vi "Read Region.vi"(8 "error in (no error)":errorcluster, 11 "AWS Core in":refnum<class "Bucket.lvclass">) -> (0 "error out":errorcluster, 2 "Region":T1, 3 "AWS Core out":refnum<class "Bucket.lvclass">)   [LabVIEW 2015, in "NI_AWS_S3.lvlib" / "Bucket.lvclass"]
uses:
  Bucket.lvclass
  Core/HTTP Request/Region.ctl
  Core/HTTP Request/HTTP Request.lvclass/HTTP Request.ctl
  Core/HTTP Request/Write Region.vi
  Core/HTTP Request/Read _regionSet.vi
  Core/HTTP Request/HTTP Request.lvclass
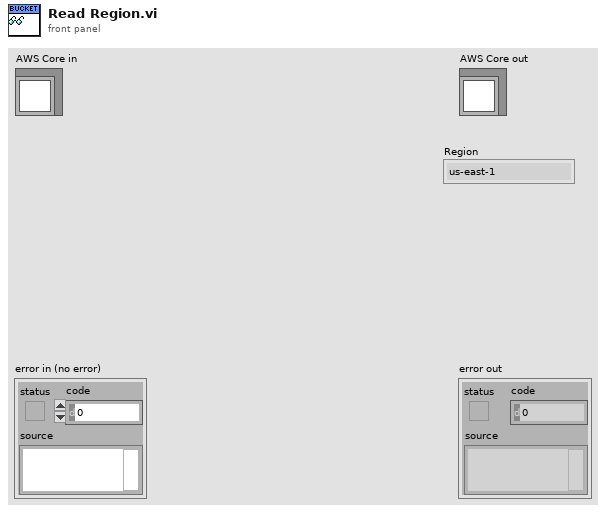
[diagram p1: front panel]
types:
  T1 = typedef "NI_AWS_Core.lvlib/HTTP Request.lvclass/Region.ctl" = enum16{"us-east-1", "us-east-2", "us-west-1", "us-west-2", "ap-northeast-1", "ap-northeast-2", "ap-southeast-1", "ap-southeast-2", "ca-central-1", "eu-central-1", "eu-west-1", "eu-west-2", "sa-east-1"}
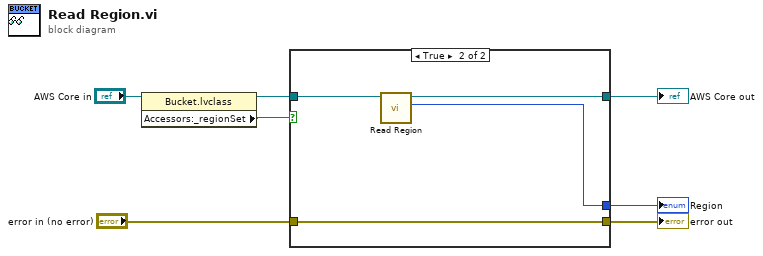
[diagram p0: block diagram]
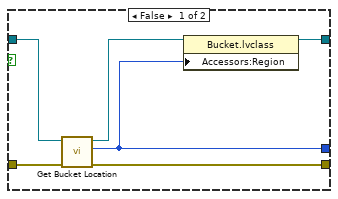
[diagram p2: hidden frame]
diagram:
  n1 = property class="Bucket.lvclass"(reference="AWS Core in") -> (reference out=w3:refnum<class "Bucket.lvclass">, "Accessors:_regionSet"=w4:bool)  [unwired: 1 in, 1 out]
  n2 = case shown="True" w4 {
    tunnel: "error in (no error)" -> [w13 w17]
    tunnel: [w12 w17] -> w5
    tunnel: [w11 w15] -> w2
    tunnel: w3 -> [w8 w16]
    tunnel: [w9 w14] -> w1
    frame False {
      n3 = call "Get Bucket Location.vi"("error in (no error)"=w13, "Bucket in"=w8) -> ("error out"=w12:errorcluster, "Location"=w9:T1, "Bucket out"=w10:refnum<class "Bucket.lvclass">)  [unwired: 7 in]
      n4 = property class="Bucket.lvclass"(reference=w10, "Accessors:Region"=w9) -> (reference out=w11:refnum<class "Bucket.lvclass">)  [unwired: 1 in, 1 out]
    }
    frame True {
      n5 = call-parent "Read Region.vi"("AWS Core in"=w16) -> ("Region"=w14:T1, "AWS Core out"=w15:refnum<class "Bucket.lvclass">)  [unwired: 8 in, 1 out]
    }
  }
  "error out" <- w5
  "AWS Core out" <- w2
  "Region" <- w1
